vi "Tab_Bool.vi"() -> ()   [LabVIEW 2020]
panel:
  in  "Tab_Bool 4":bool[](array[boolean])
  in  "Tab_Bool 3":bool[](array[boolean])
  out "Tab_Bool et Tab_Bool 3":bool[](array[boolean])
  out "Tab_Bool et Tab_Bool 2":bool[](array[boolean])
  in  "Tab_Bool 2":bool[](array[boolean])
  in  "Tab_Bool":bool[](array[boolean])
  # "ET"
  # "OU"
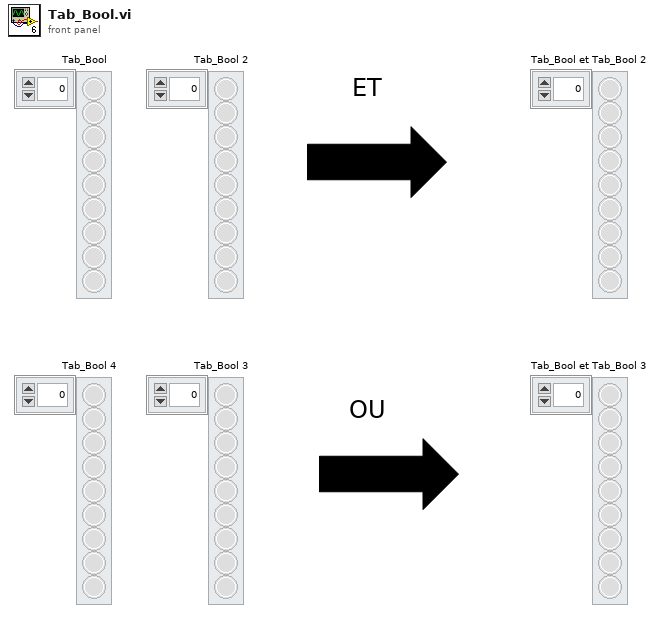
[diagram p1: front panel]
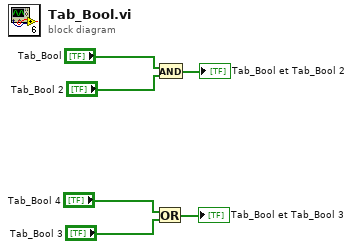
[diagram p0: block diagram]
diagram:
  n1 = Or(x="Tab_Bool 4", y="Tab_Bool 3") -> (x .or. y?=→"Tab_Bool et Tab_Bool 3":bool[])
  n2 = And(x="Tab_Bool", y="Tab_Bool 2") -> (x .and. y?=→"Tab_Bool et Tab_Bool 2":bool[])
